vi "OSC Configuration FGV.vi"(4 "error in":errorcluster, 6 "Function":enum16{"write", "read"}(ring), 7 "OSC Configuration":T1(array[cluster])=[[{"Signal Type"=enum."Sine Wave", "DC"=0.0003, "Amplitude"=0.0005, "frequency"=1.3459999999999999, "Phase"=0.0}, {"Signal Type"=enum."Sine Wave", "DC"=0.0, "Amplitude"=0.0, "frequency"=1.346, "Phase"=0.0}, {"Signal Type"=enum."Sine Wave", "DC"=0.0, "Amplitude"=0.0, "frequency"=1.346, "Phase"=0.0}, {"Signal Type"=enum."Sine Wave", "DC"=0.0, "Amplitude"=0.0, "frequency"=1.346, "Phase"=0.0}]] {"frequency" step=0.001 format="%.3p"; "Amplitude" format="%0.2p"; "DC" min=-0.99 max=0.99 format="%.2p"}) -> (0 "error out":errorcluster, 3 "OSC Configuration":T1(array[cluster])=[[{"Signal Type"=enum."Sine Wave", "DC"=0.0003, "Amplitude"=0.0005, "frequency"=1.3459999999999999, "Phase"=0.0}, {"Signal Type"=enum."Sine Wave", "DC"=0.0, "Amplitude"=0.0, "frequency"=1.346, "Phase"=0.0}, {"Signal Type"=enum."Sine Wave", "DC"=0.0, "Amplitude"=0.0, "frequency"=1.346, "Phase"=0.0}, {"Signal Type"=enum."Sine Wave", "DC"=0.0, "Amplitude"=0.0, "frequency"=1.346, "Phase"=0.0}]] {"frequency" step=0.001 format="%.3p"; "Amplitude" format="%0.2p"; "DC" min=-0.99 max=0.99 format="%.2p"})   [LabVIEW 2013]
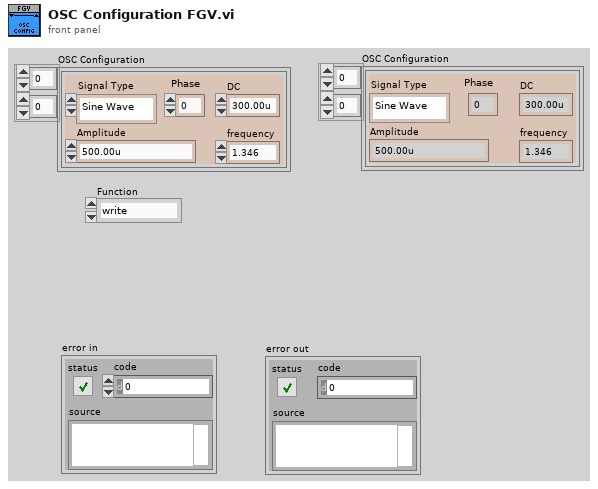
[diagram p1: front panel]
types:
  T1 = cluster{"Signal Type":enum16{"Sine Wave", "Triangle Wave", "Square Wave", "Sawtooth Wave"}, "DC":dbl, "Amplitude":dbl, "frequency":dbl, "Phase":dbl}[][]
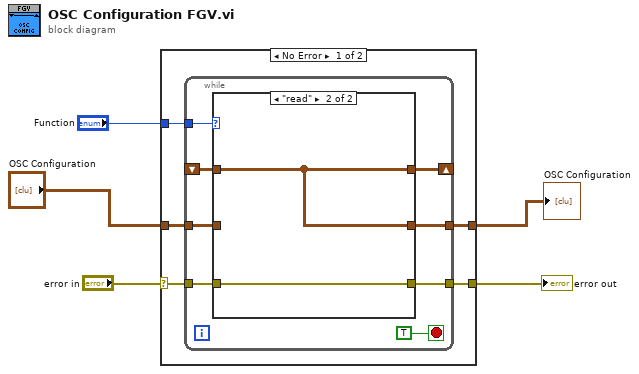
[diagram p0: block diagram]
diagram:
  n1 = case shown="No Error" "error in" {
    selector: "error in" -> [w10 w24]
    tunnel: [w9 w24] -> w4
    tunnel: "OSC Configuration" -> [w8 w23]
    tunnel: [w7 w23] -> w1
    tunnel: "Function" -> [w6 _]
    frame No Error {
      n2 = while {
        shift-right: [w12] -> _
        shift-left: _ -> [w11]
        tunnel: w10 -> [w17]
        tunnel: [w16] -> w9
        tunnel: w8 -> [w15]
        tunnel: [w14] -> w7
        tunnel: w6 -> [w13]
        stop <- TRUE stop-if-true
        n3 = case shown="\"read\"" w13 {
          tunnel: w17 -> [w19 w22]
          tunnel: [w19 w22] -> w16
          tunnel: w15 -> [w20 _]
          tunnel: [w20 w21] -> w14
          tunnel: [w20 w21] -> w12
          tunnel: w11 -> [_ w21]
          frame "write", Default {
          }
          frame "read" {
          }
        }
      }
    }
    frame Error {
    }
  }
  "error out" <- w4
  "OSC Configuration" <- w1
